vi "Keithley_2010_DCV_vs_time.vi"() -> ()   [LabVIEW 2017]
uses:
  ~~wafer_mapping_automation~~/subvis/keithley/Keithley_2010/kei2010.llb/Keithley 2010 Reset / Preset.vi
panel:
  in  "reset/preset":bool=TRUE
  in  "Terminals":bool
  in  "Ratio":bool
  in  "reference value (volts)":dbl min=-1000000000.0 max=1000000000.0 format="%^.2e"
  in  "range value (volts)":dbl=100.0 min=0.1 max=1000.0 step=0.1 format="%.1f"
  in  "dig. filter count":dbl=10.0 min=1.0 max=100.0 step=1.0 format="%^.2e"
  in  "digital filter (off:0)":u16(ring) items=["off", "moving filter", "repeating filter"]
  in  "reference (off:0)":u16(ring) items=["off", "set reference value"]
  in  "range (auto:0)":u16(ring) items=["autorange", "set range value"]
  in  "Number Power Line Cycles":dbl=1.0 min=0.01 max=10.0 step=0.01 format="%.2f"
  in  "resolution (6.5 digits:3)":u16(ring)=3 items=["3.5 digits", "4.5 digits", "5.5 digits", "6.5 digits", "7.5 digits"]
  in  "display":u16(ring)=1 items=["off", "Display Readings", "Display Text"]
  out "error out":errorcluster
  in  "error in (no error)":errorcluster
  in  "Max Elapsed time (s)":u32
  in  "Measure Interval (ms)":u32
  out "Current":dbl caption="Measured Voltage (V)"
  in  "stop":bool
  out "XY Graph":cluster{dbl[], dbl[]}(graph)
  in  "VISA resource name":refnum<visa-resource-name>="GPIB0::24::INSTR"
  # "Keithley 2010 DMM - Sample Voltage vs Time."
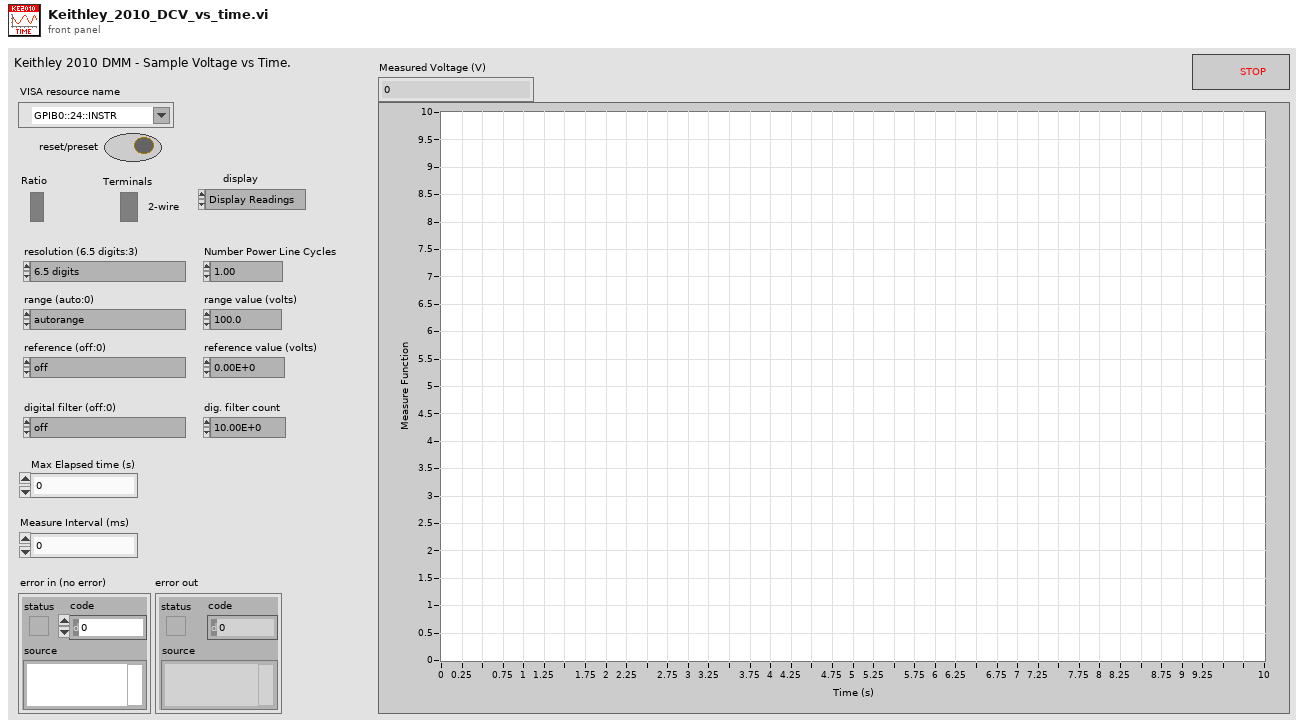
[diagram p1: front panel]
types:
  T1 = cluster{"error":bool, "code":i32, "source":string}
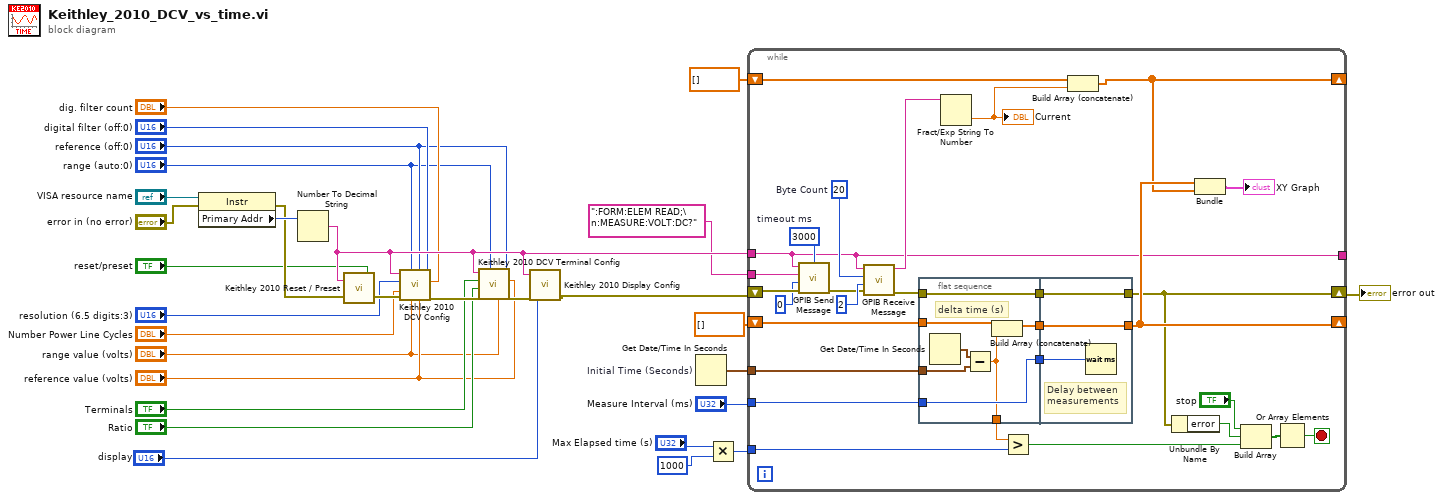
[diagram p0: block diagram]
diagram:
  n1 = property class="Instr"(reference="VISA resource name", error in="error in (no error)") -> (error out=w16:errorcluster, "Primary Addr"=w19:u16)  [unwired: 1 out]
  n2 = Number To Decimal String(number=w19) -> (decimal integer string=w15:string)  [unwired: 1 in]
  n3 = call "Keithley 2010 Reset / Preset.vi"("reset/preset"="reset/preset", "error in"=w16, "GPIB address"=w15) -> ("error out"=w17:T1)
  n4 = call "Keithley 2010 DCV Config.vi"("dig. filter count"="dig. filter count", "digital filter (off:0)"="digital filter (off:0)", "reference value (volts)"="reference value (volts)", "reference (off:0)"="reference (off:0)", "range value (volts)"="range value (volts)", "range (auto:0)"="range (auto:0)", "error in"=w17, "Number Power Line Cycles"="Number Power Line Cycles", "resolution (6.5 digits:3)"="resolution (6.5 digits:3)", "GPIB address"=w15) -> ("error out"=w18:T1)  [unwired: 1 in]
  n5 = call "Keithley 2010 DCV Terminal Config.vi"("reference value (volts)"="reference value (volts)", "reference (off:0)"="reference (off:0)", "range value (volts)"="range value (volts)", "range (auto:0)"="range (auto:0)", "error in"=w18, "Ratio"="Ratio", "Terminals"="Terminals", "GPIB address"=w15) -> ("error out"=w23:T1)  [unwired: 1 in]
  n6 = call "Keithley 2010 Display Config.vi"("error in"=w23, "display \n(Display Readings:1)"="display", "GPIB address"=w15) -> ("error out"=w22:T1)  [unwired: 2 in]
  n7 = Get Date/Time In Seconds "Initial Time (Seconds)"() -> (seconds since 1Jan1904=w30:timestamp)
  n8 = Multiply(x="Max Elapsed time (s)", y=u32 1000) -> (x*y=w24:u32)
  n9 = while {
    shift-right: [w49] -> w12
    shift-left: w22 -> [w46]
    tunnel: w30 -> [w34]
    shift-right: [w56] -> _
    shift-left: dbl[] [] -> [w33]
    shift-right: [w55] -> _
    shift-left: dbl[] [] -> [w59]
    tunnel: "Measure Interval (ms)" -> [w48]
    tunnel: w24 -> [w53]
    tunnel: [w38] -> _
    tunnel: w15 -> [w38]
    tunnel: ":FORM:ELEM READ;\n:MEASURE:VOLT:DC?" -> [w37]
    stop <- w58 stop-if-true
    w39 = u32 3000  # timeout ms
    w44 = 20  # Byte Count
    n10 = call "GPIB Send Message.vi"("timeout ms"=w39, "address string"=w38, "write buffer"=w37, "write mode (set END:0)"=0, "error in"=w46) -> ("error out"=w43:T1)  [unwired: 2 in, 2 out]
    n11 = call "GPIB Receive Message.vi"("address string"=w38, "byte count"=w44, "read mode"=2, "error in"=w43) -> ("read buffer"=w41:string, "error out"=w42:T1)  [unwired: 3 in, 1 out]
    n12 = flat-sequence {
      tunnel: w42 -> [w65]
      tunnel: w48 -> [w66]
      tunnel: [w66] -> w36
      tunnel: [w65] -> w35
      tunnel: w34 -> [w63]
      tunnel: w33 -> [w62]
      tunnel: [w61] -> w32
      tunnel: [w60] -> w31
      tunnel: [w69] -> w56
      tunnel: [w67] -> w49
      tunnel: w36 -> [w68]
      tunnel: w35 -> [w67]
      tunnel: w32 -> [w69]
      frame #0 {
        # "delta time (s)"
        n13 = Get Date/Time In Seconds() -> (seconds since 1Jan1904=w64:timestamp)
        n14 = Subtract(x=w64, y=w63) -> (x-y=w60:dbl)
        n15 = Build Array (concatenate)(w62, w60) -> (w61:dbl[])
      }
      frame #1 {
        # "Delay between\nmeasurements"
        n16 = Wait (ms)(milliseconds to wait=w68) -> ()  [unwired: 1 out]
      }
    }
    n17 = Fract/Exp String To Number(string=w41) -> (number=w47:dbl)  [unwired: 3 in, 1 out]
    "Current" <- w47
    n18 = Greater?(x=w31, y=w53) -> (0:w50:bool)
    n19 = Build Array (concatenate)(w59, w47) -> (w55:dbl[])
    n20 = Unbundle By Name(w49) -> ("error"=w51:bool)
    n21 = Bundle(w56, w55) -> (→"XY Graph":cluster{dbl[], dbl[]})  [unwired: 1 in]
    n22 = Build Array("stop", w51, w50) -> (w57:bool[])
    n23 = Or Array Elements(Boolean array=w57) -> (logical OR=w58:bool)
  }
  "error out" <- w12
